vi "Do on Error.vi"(8 "error in (no error)":errorcluster, 11 "LAC Error Logger in":refnum<class "LAC Error Logger.lvclass">) -> ()   [LabVIEW 2018, in "Assert API Components.lvlib" / "Log Assert Core.lvlib" / "LAC Error Logger.lvclass"]
doc: "Dynamic dispatch vi to be overriden by file or debug UI - takes the action to pass the error and handle it as required."
uses:
  LAC Error Logger.lvclass
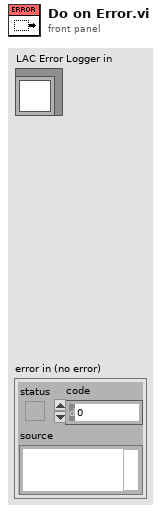
[diagram p1: front panel]
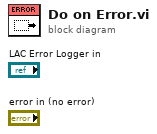
[diagram p0: block diagram]
diagram:
